vi "Open.vi"(8 "error in":errorcluster, 11 "Vaisala in":refnum<class "Vaisala.lvclass">) -> (0 "error out":errorcluster, 3 "Vaisala out":refnum<class "Vaisala.lvclass">)   [LabVIEW 2014, in "Vaisala.lvclass"]
uses:
  Vaisala.lvclass
  Vaisala.lvclass/Vaisala.ctl
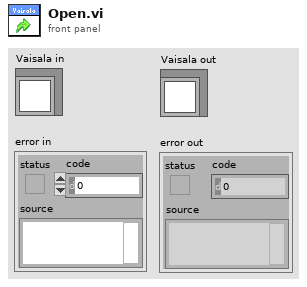
[diagram p1: front panel]
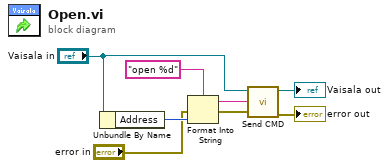
[diagram p0: block diagram]
diagram:
  n1 = Unbundle By Name("Vaisala in") -> ("Address"=w4:u8)
  n2 = Format Into String(format string="open %d", error in="error in", w4) -> (resulting string=w3:string, error out=w1:errorcluster)  [unwired: 1 in]
  n3 = call-dynamic "Send CMD.vi"("error in"=w1, "CMD In"=w3, "Vaisala in"="Vaisala in") -> ("error out"=→"error out":errorcluster, "Vaisala out"=→"Vaisala out":refnum<class "Vaisala.lvclass">)  [unwired: 7 in]
